vi "Create Enum Paths.vi"(8 "error in (no error)":errorcluster, 9 "Enumeration Name":string, 11 "LV-Protoc in":refnum<class "LV-Protoc.lvclass">) -> (0 "error out":errorcluster, 3 "LV-Protoc out":refnum<class "LV-Protoc.lvclass">, 4 "Enumeration Paths":T1)   [LabVIEW 2020, in "LV-Protoc.lvlib" / "LV-Protoc.lvclass"]
uses:
  LV-Protoc.lvclass
  Enumeration Paths.ctl
  LV-Protoc.lvclass/LV-Protoc.ctl
  LV-Protoc.lvlib
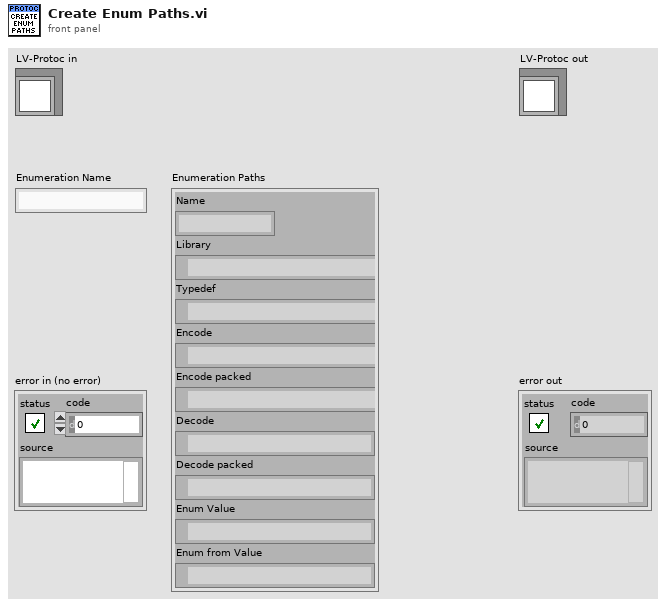
[diagram p1: front panel]
types:
  T1 = typedef "LV-Protoc.lvlib/Enumeration Paths.ctl" = cluster{"Name":string, "Library":path, "Typedef":path, "Encode":path, "Encode packed":path, "Decode":path, "Decode packed":path, "Enum Value":path, "Enum from Value":path}
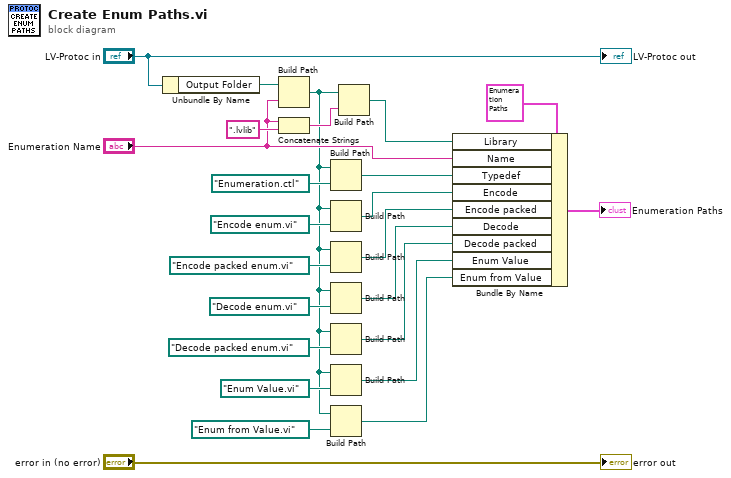
[diagram p0: block diagram]
diagram:
  n1 = Unbundle By Name("LV-Protoc in") -> ("Output Folder"=w24:path)
  n2 = Build Path(base path=w24, name or relative path="Enumeration Name") -> (appended path=w3:path)
  n3 = Concatenate Strings("Enumeration Name", ".lvlib" ("string")) -> (w22:string)
  n4 = Build Path(base path=w3, name or relative path=path "Enumeration.ctl") -> (appended path=w15:path)
  n5 = Build Path(base path=w3, name or relative path=path "Encode enum.vi") -> (appended path=w12:path)
  n6 = Build Path(base path=w3, name or relative path=path "Encode packed enum.vi") -> (appended path=w11:path)
  n7 = Build Path(base path=w3, name or relative path=path "Decode enum.vi") -> (appended path=w7:path)
  n8 = Build Path(base path=w3, name or relative path=path "Decode packed enum.vi") -> (appended path=w6:path)
  n9 = Build Path(base path=w3, name or relative path=path "Enum Value.vi") -> (appended path=w2:path)
  n10 = Build Path(base path=w3, name or relative path=path "Enum from Value.vi") -> (appended path=w1:path)
  n11 = Build Path(base path=w3, name or relative path=w22) -> (appended path=w14:path)
  n12 = Bundle By Name(cluster=T1 {"Name"="", "Library"=path "", "Typedef"=path "", "Encode"=path "", "Encode packed"=path "", "Decode"=path "", "Decode packed"=path "", "Enum Value"=path "", "Enum from Value"=path ""} ("Built Enumeration"), "Library"=w14, "Name"="Enumeration Name", "Typedef"=w15, "Encode"=w12, "Encode packed"=w11, "Decode"=w7, "Decode packed"=w6, "Enum Value"=w2, "Enum from Value"=w1) -> (→"Enumeration Paths":T1)
  "error out" <- "error in (no error)"
  "LV-Protoc out" <- "LV-Protoc in"
